vi "List Tables.vi"(8 "error in (no error)":errorcluster, 11 "database in":path=path "C:/labview/sqlite_dbManager/test database/chinook.db") -> (0 "error out":errorcluster, 2 "Tables":string[](array[string]))   [LabVIEW 2020, in "sqlite3.lvlib"]
uses:
  sqlite3.lvlib
  sqlite/VIs/open v2.vi
  sqlite/VIs/prepare v2.vi
  sqlite/VIs/step.vi
  sqlite/VIs/column count.vi
  compound/Column.vi
  compound/Resolve Result Type.vi
  sqlite/VIs/finalize.vi
  sqlite/VIs/close v2.vi
  sqlite/subvi/Error Converter (ErrCode or Status).vi
  sqlite/VIs/column text.vi
  sqlite/VIs/column bytes.vi
  sqlite/VIs/column blob.vi
  utilities/MoveBlock.vi
  sqlite/VIs/column type.vi
  sqlite/VIs/errstr.vi
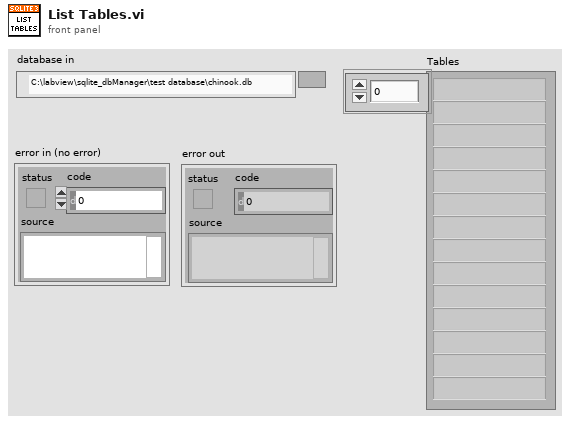
[diagram p1: front panel]
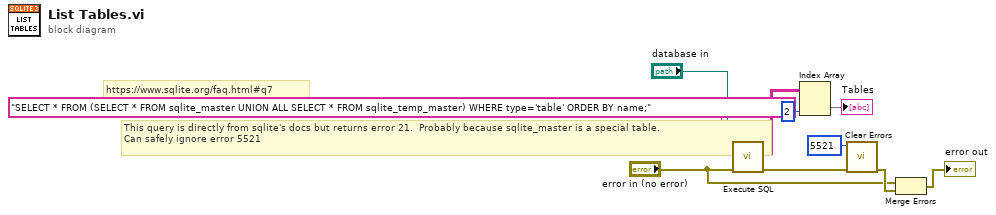
[diagram p0: block diagram]
diagram:
  # "This query is directly from sqlite's docs but returns error 21.  Probably because sqlite_master is a special table.\nCan safely ignore error 5521"
  # "https://www.sqlite.org/faq.html#q7"
  n1 = call "Execute SQL.vi"("error in (no error)"="error in (no error)", "sql (string)"="SELECT * FROM (SELECT * FROM sqlite_master UNION ALL SELECT * FROM sqlite_temp_master) WHERE type='table' ORDER BY name;", "database in"="database in") -> ("error out"=w5:errorcluster, "Query Result"=w10:string[][])  [unwired: 7 in]
  n2 = Index Array(array=w10, index (col)=2 ("index (row)")) -> (element=→"Tables":string[])  [unwired: 1 in]
  n3 = call <vilib>:"Clear Errors.vi"("error in (no error)"=w5, "specific error code to clear (0: all)"=5521) -> ("error out"=w4:errorcluster)  [unwired: 4 in, 1 out]
  n4 = Merge Errors("error in (no error)", w4) -> (→"error out":errorcluster)
